vi "Setup.vi"(11 "Queue Transport in":refnum<class "Queue Transport.lvclass">) -> (0 "Error out":errorcluster, 3 "Queue Transport out":refnum<class "Queue Transport.lvclass">)   [LabVIEW 2020, in "jettl.lvlib" / "Queue Transport.lvlib" / "Queue Transport.lvclass"]
uses:
  Queue Transport.lvclass
  Msg/Msg.lvclass
  Queue Transport.lvclass/Queue Transport.ctl
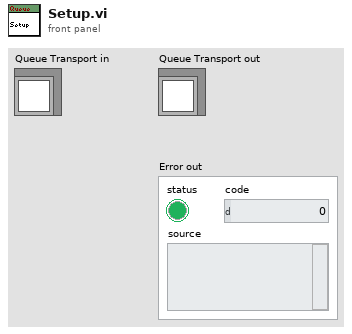
[diagram p1: front panel]
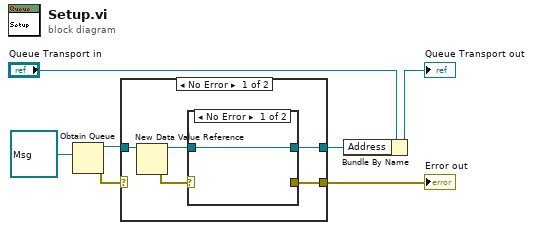
[diagram p0: block diagram]
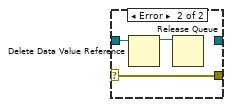
[diagram p2: hidden frame]
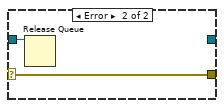
[diagram p3: hidden frame]
diagram:
  n1 = Obtain Queue(element data type=refnum<class "Msg.lvclass"> refnum ("Msg")) -> (queue out=w2:refnum<queue>, error out=w4:errorcluster)  [unwired: 4 in, 1 out]
  n2 = case shown="No Error" w4 {
    selector: w4 -> [_ w18]
    tunnel: [w10 w18] -> w3
    tunnel: w2 -> [w12 w17]
    tunnel: [w8 _] -> w1
    frame No Error {
      n3 = New Data Value Reference(data value=w12) -> (data value reference=w9:refnum<data-value>, error out=w11:errorcluster)  [unwired: 1 in]
      n4 = case shown="No Error" w11 {
        selector: w11 -> [_ w16]
        tunnel: [_ w16] -> w10
        tunnel: w9 -> [w13 w15]
        tunnel: [w13 _] -> w8
        frame No Error {
        }
        frame Error {
          n5 = Delete Data Value Reference(data value reference=w15) -> (data value=w14:refnum<queue>)  [unwired: 1 in, 1 out]
          n6 = Release Queue(queue=w14) -> ()  [unwired: 2 in, 3 out]
        }
      }
    }
    frame Error {
      n7 = Release Queue(queue=w17) -> ()  [unwired: 2 in, 3 out]
    }
  }
  "Error out" <- w3
  n8 = Bundle By Name(cluster="Queue Transport in", "Address"=w1) -> (→"Queue Transport out":refnum<class "Queue Transport.lvclass">)
